vi "Build Wiring Spec.vi"(8 "error in (no error)":errorcluster, 11 "CS++Actor in":refnum<class "CS++Actor.lvclass">) -> (0 "error out":errorcluster, 2 "Wiring Spec":T1, 3 "CS++Actor out":refnum<class "CS++Actor.lvclass">)   [LabVIEW 2016, in "CS++Actor.lvlib" / "CS++Actor.lvclass"]
doc: "Create the Wiring Spec of the original public Vi."
uses:
  CS++Actor.lvclass
  CS++Actor.lvclass/CS++Actor.ctl
  <vilib>/Utility/Data Type/NI_Data Type.lvlib
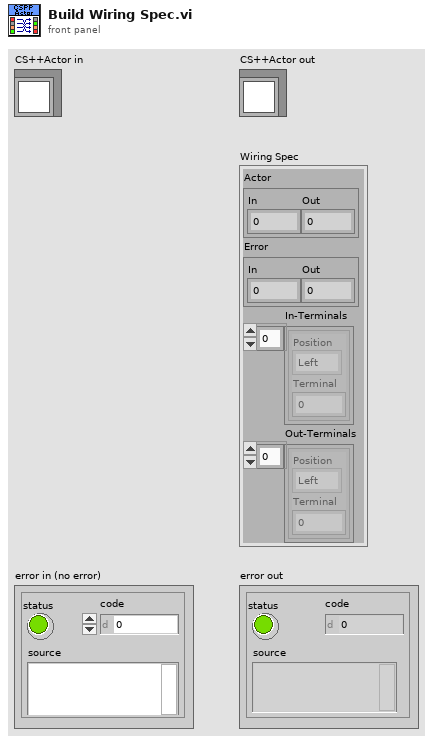
[diagram p1: front panel]
types:
  T1 = cluster{"Actor":cluster{"In":i32, "Out":i32}, "Error":cluster{"In":i32, "Out":i32}, "In-Terminals":cluster{"Position":enum16{"Left", "Top", "Bottom", "Right"}, "Terminal":i32}[], "Out-Terminals":cluster{"Position":enum16{"Left", "Top", "Bottom", "Right"}, "Terminal":i32}[]}
  T2 = cluster{"Actor":cluster{"In":i32, "Out":i32}, "Error":cluster{"In":i32, "Out":i32}, "Left":cluster{"Position":i16, "Terminal":i32}[], "Bottom":cluster{"Position":i16, "Terminal":i32}[], "Right":cluster{"Position":i16, "Terminal":i32}[], "Top":cluster{"Position":i16, "Terminal":i32}[]}
  T3 = enum16{"Invalid Wire Rule", "Required", "Recommended", "Optional", "Dynamic Dispatch"}[]
  T4 = typedef "LVRectTypeDef.ctl" = cluster{"Left":i16, "Top":i16, "Right":i16, "Bottom":i16}
  T5 = cluster{"Position":enum16{"Left", "Top", "Bottom", "Right"}, "Terminal":i32}
  T6 = cluster{"Position":enum16{"Left", "Top", "Bottom", "Right"}, "Terminal":i32}[]
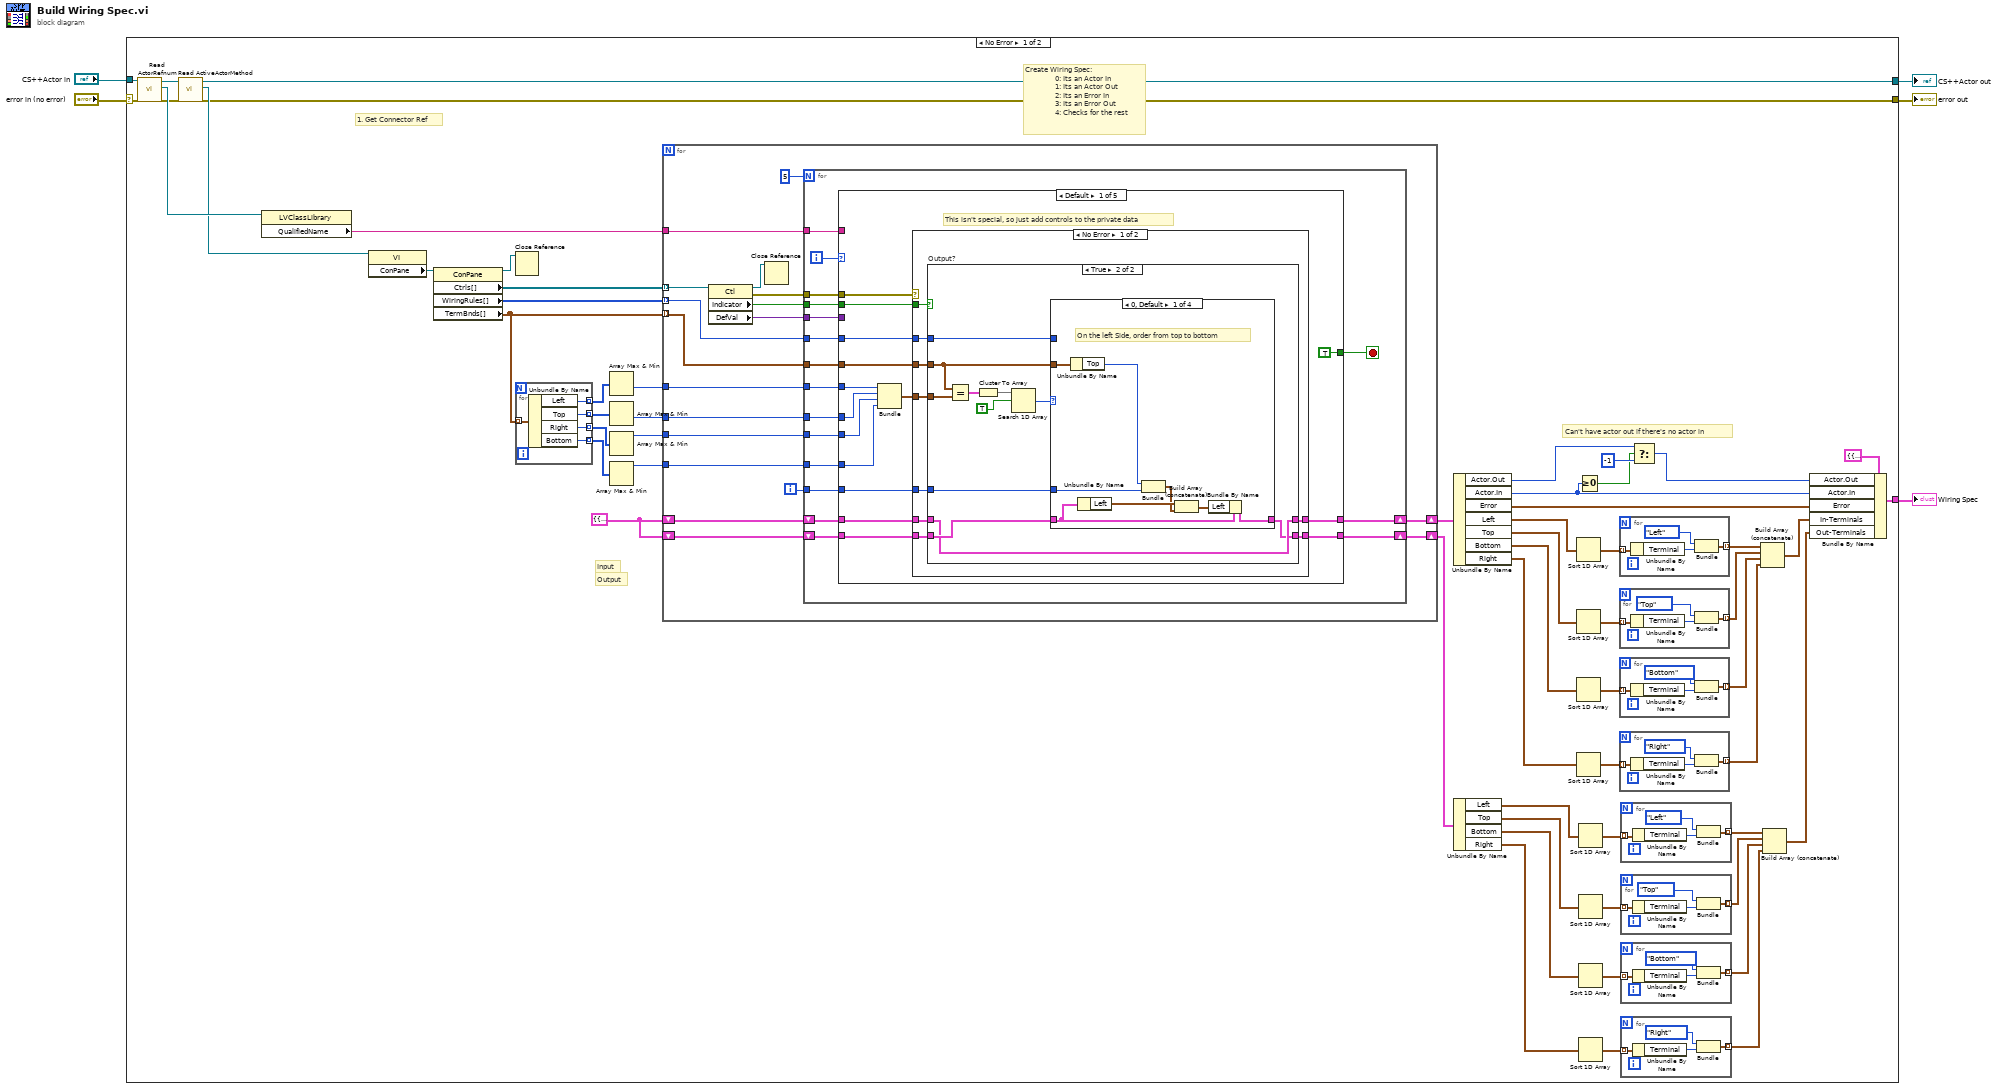
[diagram p0: block diagram]
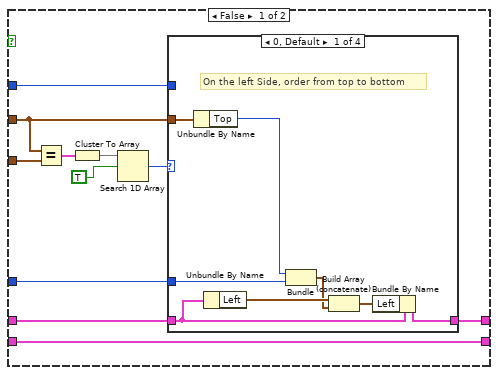
[diagram p2: hidden frame]
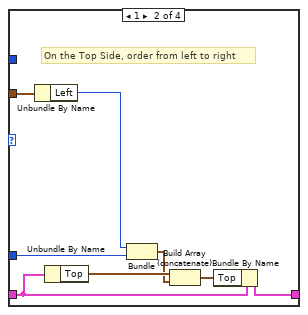
[diagram p3: hidden frame]
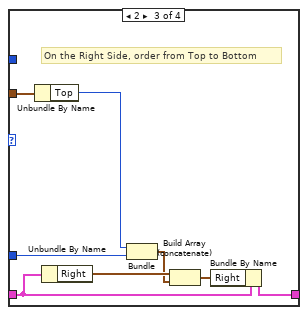
[diagram p4: hidden frame]
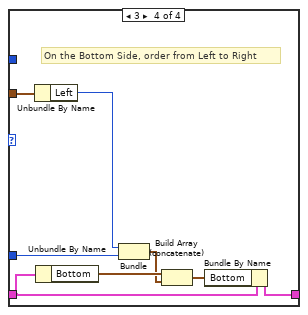
[diagram p5: hidden frame]
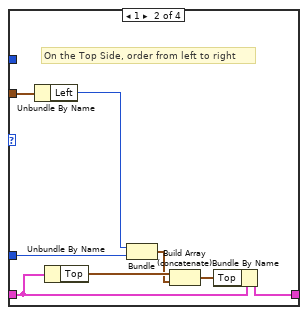
[diagram p6: hidden frame]
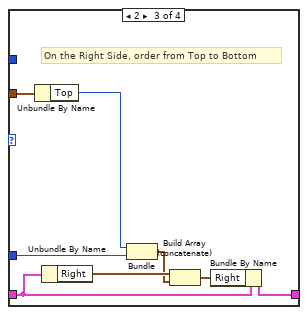
[diagram p7: hidden frame]
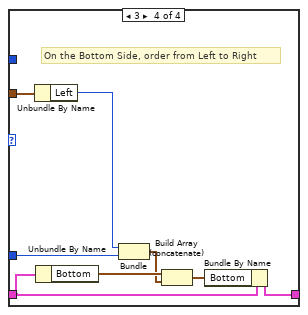
[diagram p8: hidden frame]
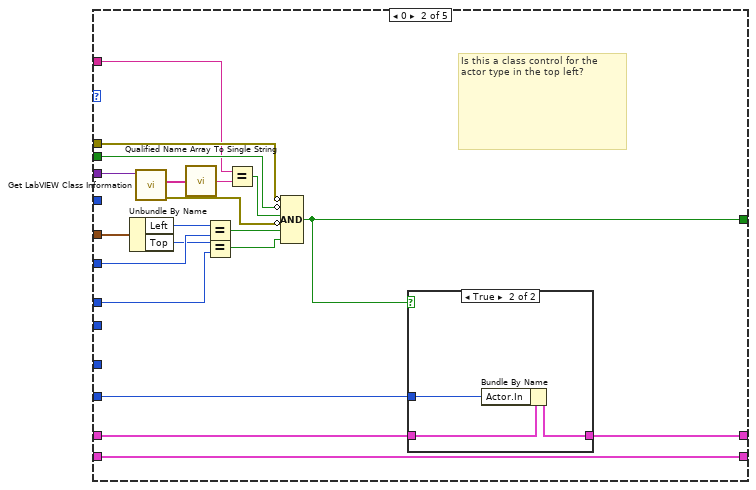
[diagram p10: hidden frame]
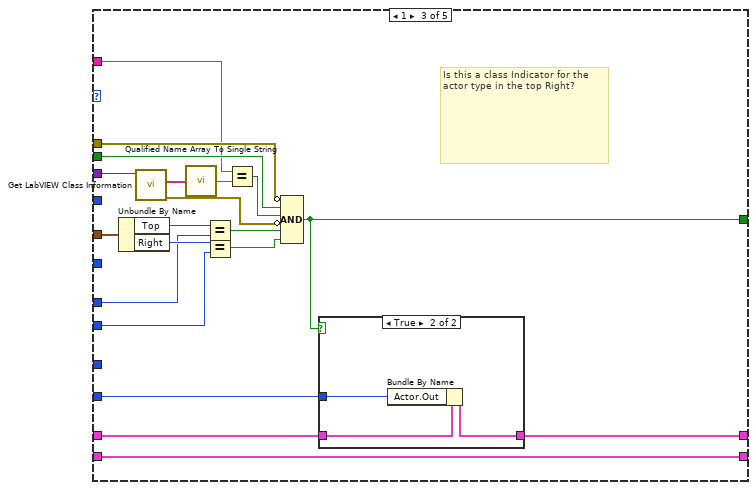
[diagram p12: hidden frame]
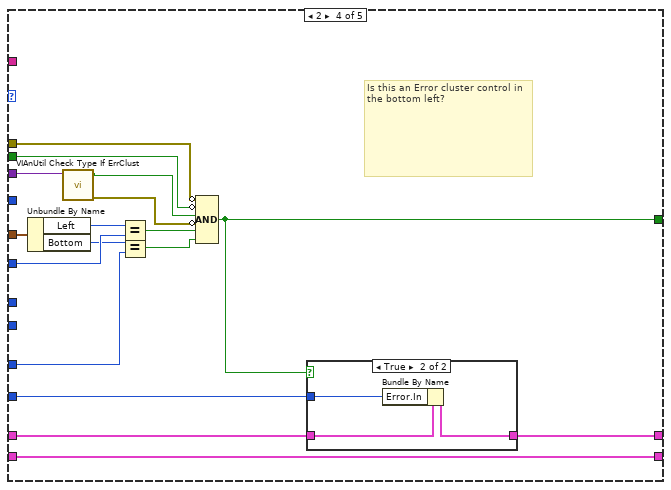
[diagram p14: hidden frame]
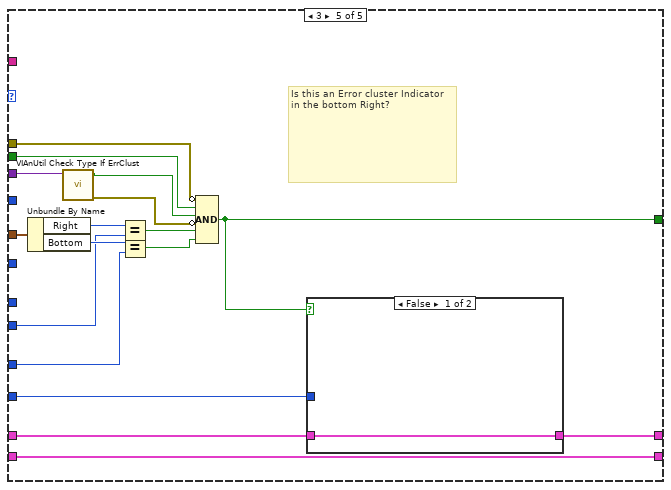
[diagram p16: hidden frame]
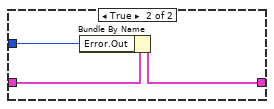
[diagram p17: hidden frame]
diagram:
  n1 = case shown="No Error" "error in (no error)" {
    selector: "error in (no error)" -> [w21 w339]
    tunnel: [w42 _] -> w5
    tunnel: "CS++Actor in" -> [w28 w340]
    tunnel: [w23 w339] -> w3
    tunnel: [w22 w340] -> w2
    frame No Error {
      w20 = T2 {"Actor"={"In"=-1, "Out"=-1}, "Error"={"In"=-1, "Out"=-1}, "Left"=[], "Bottom"=[], "Right"=[], "Top"=[]}
      # "Output"
      # "Input"
      # "Create Wiring Spec:\n               0: Its an Actor In\n               1: Its an Actor Out\n               2: Its an Error In\n               3: Its an Error Out \n               4: Checks for the rest"
      # "1. Get Connector Ref"
      # "Can't have actor out if there's no actor in"
      n2 = call "Read ActorRefnum.vi"("error in (no error)"=w21, "CS++Actor in"=w28) -> ("error out"=w25:errorcluster, "ActorRefnum"=w27:refnum<vi>, "CS++Actor out"=w26:refnum<class "CS++Actor.lvclass">)  [unwired: 7 in]
      n3 = call "Read ActiveActorMethod.vi"("error in (no error)"=w25, "CS++Actor in"=w26) -> ("error out"=w23:errorcluster, "ActiveActorMethod"=w24:refnum<vi>, "CS++Actor out"=w22:refnum<class "CS++Actor.lvclass">)  [unwired: 7 in]
      n4 = property class="LVClassLibrary"(reference=w27) -> ("QualifiedName"=w29:string)  [unwired: 1 in, 2 out]
      n5 = property class="VI"(reference=w24) -> ("ConPane"=w64:refnum<vi>)  [unwired: 1 in, 2 out]
      n6 = property class="ConPane"(reference=w64) -> (reference out=w53:refnum<vi>, "Ctrls[]"=w63:refnum<vi>[], "WiringRules[]"=w41:T3, "TermBnds[]"=w62:T4[])  [unwired: 1 in, 1 out]
      n7 = Close Reference(reference=w53) -> ()  [unwired: 1 in, 1 out]
      n8 = for {
        tunnel: w62 -> [w69] mode=indexing
        tunnel: [w68] -> w61 mode=indexing
        tunnel: [w67] -> w60 mode=indexing
        tunnel: [w66] -> w59 mode=indexing
        tunnel: [w65] -> w58 mode=indexing
        n9 = Unbundle By Name(w69) -> ("Left"=w68:i16, "Top"=w67:i16, "Right"=w66:i16, "Bottom"=w65:i16)
      }
      n10 = Array Max & Min(array=w61) -> (min value=w57:i16)  [unwired: 3 out]
      n11 = Array Max & Min(array=w60) -> (min value=w56:i16)  [unwired: 3 out]
      n12 = Array Max & Min(array=w59) -> (max value=w55:i16)  [unwired: 3 out]
      n13 = Array Max & Min(array=w58) -> (max value=w54:i16)  [unwired: 3 out]
      n14 = for {
        tunnel: w63 -> [w87] mode=indexing
        tunnel: w62 -> [w85] mode=indexing
        tunnel: w57 -> [w84]
        tunnel: w56 -> [w83]
        tunnel: w55 -> [w76]
        tunnel: w54 -> [w77]
        tunnel: w29 -> [w79]
        shift-right: [w73] -> w52
        shift-left: w20 -> [w74]
        tunnel: w41 -> [w72] mode=indexing
        shift-right: [w70] -> w6
        shift-left: w20 -> [w71]
        i -> [w78]
        # "Find Top Left, Bottom left controls AND\nTop Right and bottom right Indicators"
        n15 = property class="Ctl"(reference=w87) -> (reference out=w75:refnum<vi>, error out=w82:errorcluster, "Indicator"=w81:bool, "DefVal"=w80:variant)  [unwired: 1 in]
        n16 = Close Reference(reference=w75) -> ()  [unwired: 1 in, 1 out]
        n17 = for {
          N: 5 -> [_]
          tunnel: w85 -> [w103]
          shift-right: [w94] -> w73
          shift-left: w74 -> [w102]
          tunnel: w84 -> [w101]
          tunnel: w83 -> [w100]
          tunnel: w82 -> [w99]
          tunnel: w81 -> [w98]
          tunnel: w80 -> [w97]
          tunnel: w79 -> [w96]
          tunnel: w78 -> [w95]
          tunnel: w77 -> [w93]
          tunnel: w76 -> [w92]
          tunnel: w72 -> [w90]
          shift-right: [w88] -> w70
          shift-left: w71 -> [w89]
          i -> [w104]
          stop <- w91 stop-if-true
          n18 = case shown="Default" w104 {
            tunnel: w103 -> [w115 w236 w260 w281 w302]
            tunnel: w102 -> [w119 w221 w247 w267 w288]
            tunnel: w101 -> [w114 w234 _ w279 _]
            tunnel: w100 -> [w113 w232 w245 _ _]
            tunnel: w99 -> [w108 w231 w257 w277 w299]
            tunnel: w98 -> [w107 w230 w256 w276 w298]
            tunnel: w97 -> [_ w226 w252 w272 w294]
            tunnel: w96 -> [_ w223 w249 _ _]
            tunnel: w95 -> [w117 w220 w246 w273 w295]
            tunnel: [w118 w218 w242 w266 w287] -> w94
            tunnel: w93 -> [w111 _ _ w269 w291]
            tunnel: w92 -> [w112 _ w244 _ w290]
            tunnel: [TRUE w219 w243 w268 w289] -> w91
            tunnel: w90 -> [w109 _ _ _ _]
            tunnel: w89 -> [w106 w217 w241 w265 w286]
            tunnel: [w105 w217 w241 w265 w286] -> w88
            frame Default {
              # "This isn't special, so just add controls to the private data"
              n19 = Bundle(w114, w113, w112, w111) -> (w110:cluster{i16, i16, i16, i16})  [unwired: 1 in]
              n20 = case shown="No Error" w108 {
                tunnel: w119 -> [w128 w216]
                tunnel: [w127 w216] -> w118
                tunnel: w107 -> [w126 _]
                tunnel: w117 -> [w125 _]
                tunnel: w115 -> [w124 _]
                tunnel: w110 -> [w123 _]
                tunnel: w109 -> [w122 _]
                tunnel: w106 -> [w121 w215]
                tunnel: [w120 w215] -> w105
                frame No Error {
                  n21 = case "Output?" shown="True" w126 {
                    tunnel: w128 -> [w133 w173]
                    tunnel: [w131 w173] -> w127
                    tunnel: w125 -> [w132 w176]
                    tunnel: w124 -> [w134 w177]
                    tunnel: w123 -> [w139 w182]
                    tunnel: w122 -> [w130 w175]
                    tunnel: w121 -> [w129 w174]
                    tunnel: [w129 w172] -> w120
                    frame False {
                      n22 = Equal?(x=w134, y=w139) -> (x = y?=w138:cluster{bool, bool, bool, bool})
                      n23 = Cluster To Array(cluster=w138) -> (array=w137:bool[])
                      n24 = Search 1D Array(1D array=w137, element=TRUE) -> (index of element=w135:i32)  [unwired: 1 in]
                      n25 = case shown="0, Default" w135 {
                        tunnel: w134 -> [w147 w155 w163 w171]
                        tunnel: w133 -> [w144 w152 w160 w168]
                        tunnel: w132 -> [w145 w153 w161 w169]
                        tunnel: [w141 w149 w157 w165] -> w131
                        tunnel: w130 -> [_ _ _ _]
                        frame 0, Default {
                          # "On the left Side, order from top to bottom"
                          n26 = Unbundle By Name(w147) -> ("Top"=w146:i16)
                          n27 = Unbundle By Name(w144) -> ("Left"=w143:cluster{"Position":i16, "Terminal":i32}[])
                          n28 = Bundle("Top"=w146, w145) -> (w142:cluster{"Top":i16, i32})  [unwired: 1 in]
                          n29 = Build Array (concatenate)(w143, w142) -> (w140:cluster{"Top":i16, "Terminal":i32}[])
                          n30 = Bundle By Name(cluster=w144, "Left"=w140) -> (w141:T2)
                        }
                        frame 1 {
                          # "On the Top Side, order from left to right"
                          n31 = Unbundle By Name(w155) -> ("Left"=w154:i16)
                          n32 = Unbundle By Name(w152) -> ("Top"=w151:cluster{"Position":i16, "Terminal":i32}[])
                          n33 = Bundle("Left"=w154, w153) -> (w150:cluster{"Left":i16, i32})  [unwired: 1 in]
                          n34 = Build Array (concatenate)(w151, w150) -> (w148:cluster{"Left":i16, "Terminal":i32}[])
                          n35 = Bundle By Name(cluster=w152, "Top"=w148) -> (w149:T2)
                        }
                        frame 2 {
                          # "On the Right Side, order from Top to Bottom"
                          n36 = Unbundle By Name(w163) -> ("Top"=w162:i16)
                          n37 = Unbundle By Name(w160) -> ("Right"=w159:cluster{"Position":i16, "Terminal":i32}[])
                          n38 = Bundle("Top"=w162, w161) -> (w158:cluster{"Top":i16, i32})  [unwired: 1 in]
                          n39 = Build Array (concatenate)(w159, w158) -> (w156:cluster{"Top":i16, "Terminal":i32}[])
                          n40 = Bundle By Name(cluster=w160, "Right"=w156) -> (w157:T2)
                        }
                        frame 3 {
                          # "On the Bottom Side, order from Left to Right"
                          n41 = Unbundle By Name(w171) -> ("Left"=w170:i16)
                          n42 = Unbundle By Name(w168) -> ("Bottom"=w167:cluster{"Position":i16, "Terminal":i32}[])
                          n43 = Bundle("Left"=w170, w169) -> (w166:cluster{"Left":i16, i32})  [unwired: 1 in]
                          n44 = Build Array (concatenate)(w167, w166) -> (w164:cluster{"Left":i16, "Terminal":i32}[])
                          n45 = Bundle By Name(cluster=w168, "Bottom"=w164) -> (w165:T2)
                        }
                      }
                    }
                    frame True {
                      n46 = Equal?(x=w177, y=w182) -> (x = y?=w181:cluster{bool, bool, bool, bool})
                      n47 = Cluster To Array(cluster=w181) -> (array=w180:bool[])
                      n48 = Search 1D Array(1D array=w180, element=TRUE) -> (index of element=w178:i32)  [unwired: 1 in]
                      n49 = case shown="0, Default" w178 {
                        tunnel: w177 -> [w190 w198 w206 w214]
                        tunnel: w174 -> [w187 w195 w203 w211]
                        tunnel: w176 -> [w188 w196 w204 w212]
                        tunnel: [w184 w192 w200 w208] -> w172
                        tunnel: w175 -> [_ _ _ _]
                        frame 0, Default {
                          # "On the left Side, order from top to bottom"
                          n50 = Unbundle By Name(w190) -> ("Top"=w189:i16)
                          n51 = Unbundle By Name(w187) -> ("Left"=w186:cluster{"Position":i16, "Terminal":i32}[])
                          n52 = Bundle("Top"=w189, w188) -> (w185:cluster{"Top":i16, i32})  [unwired: 1 in]
                          n53 = Build Array (concatenate)(w186, w185) -> (w183:cluster{"Top":i16, "Terminal":i32}[])
                          n54 = Bundle By Name(cluster=w187, "Left"=w183) -> (w184:T2)
                        }
                        frame 1 {
                          # "On the Top Side, order from left to right"
                          n55 = Unbundle By Name(w198) -> ("Left"=w197:i16)
                          n56 = Unbundle By Name(w195) -> ("Top"=w194:cluster{"Position":i16, "Terminal":i32}[])
                          n57 = Bundle("Left"=w197, w196) -> (w193:cluster{"Left":i16, i32})  [unwired: 1 in]
                          n58 = Build Array (concatenate)(w194, w193) -> (w191:cluster{"Left":i16, "Terminal":i32}[])
                          n59 = Bundle By Name(cluster=w195, "Top"=w191) -> (w192:T2)
                        }
                        frame 2 {
                          # "On the Right Side, order from Top to Bottom"
                          n60 = Unbundle By Name(w206) -> ("Top"=w205:i16)
                          n61 = Unbundle By Name(w203) -> ("Right"=w202:cluster{"Position":i16, "Terminal":i32}[])
                          n62 = Bundle("Top"=w205, w204) -> (w201:cluster{"Top":i16, i32})  [unwired: 1 in]
                          n63 = Build Array (concatenate)(w202, w201) -> (w199:cluster{"Top":i16, "Terminal":i32}[])
                          n64 = Bundle By Name(cluster=w203, "Right"=w199) -> (w200:T2)
                        }
                        frame 3 {
                          # "On the Bottom Side, order from Left to Right"
                          n65 = Unbundle By Name(w214) -> ("Left"=w213:i16)
                          n66 = Unbundle By Name(w211) -> ("Bottom"=w210:cluster{"Position":i16, "Terminal":i32}[])
                          n67 = Bundle("Left"=w213, w212) -> (w209:cluster{"Left":i16, i32})  [unwired: 1 in]
                          n68 = Build Array (concatenate)(w210, w209) -> (w207:cluster{"Left":i16, "Terminal":i32}[])
                          n69 = Bundle By Name(cluster=w211, "Bottom"=w207) -> (w208:T2)
                        }
                      }
                    }
                  }
                }
                frame Error {
                }
              }
            }
            frame 0 {
              # "Is this a class control for the actor type in the top left?"
              # "Top Left Actor Class Ctrl?"
              n70 = Unbundle By Name(w236) -> ("Left"=w235:i16, "Top"=w233:i16)
              n71 = call <vilib>:"Get LabVIEW Class Information.vi"("Variant"=w226) -> ("error out"=w225:errorcluster, "Qualified LabVIEW Class Name"=w227:string[])  [unwired: 8 in, 1 out]
              n72 = call <vilib>:"Qualified Name Array To Single String.vi"("Fully Qualified Array"=w227) -> ("Fully Qualified String"=w224:string)
              n73 = Equal?(x=w235, y=w234) -> (x = y?=w229:bool)
              n74 = Equal?(x=w233, y=w232) -> (x = y?=w228:bool)
              n75 = Equal?(x=w223, y=w224) -> (x = y?=w222:bool)
              n76 = Compound Arithmetic op=AND(invert w231, invert w230, w222, invert w225, w229, w228) -> (w219:bool)
              n77 = case shown="True" w219 {
                tunnel: w221 -> [w237 w238]
                tunnel: w220 -> [_ w239]
                tunnel: [w237 w240] -> w218
                frame False {
                }
                frame True {
                  n78 = Bundle By Name(cluster=w238, "Actor.In"=w239) -> (w240:T2)
                }
              }
            }
            frame 1 {
              # "Is this a class Indicator for the actor type in the top Right?"
              # "Top Left Actor Class Ctrl?"
              n79 = Unbundle By Name(w260) -> ("Top"=w259:i16, "Right"=w258:i16)
              n80 = call <vilib>:"Get LabVIEW Class Information.vi"("Variant"=w252) -> ("error out"=w251:errorcluster, "Qualified LabVIEW Class Name"=w253:string[])  [unwired: 8 in, 1 out]
              n81 = call <vilib>:"Qualified Name Array To Single String.vi"("Fully Qualified Array"=w253) -> ("Fully Qualified String"=w250:string)
              n82 = Equal?(x=w259, y=w245) -> (x = y?=w255:bool)
              n83 = Equal?(x=w258, y=w244) -> (x = y?=w254:bool)
              n84 = Equal?(x=w249, y=w250) -> (x = y?=w248:bool)
              n85 = Compound Arithmetic op=AND(invert w257, w256, w248, invert w251, w255, w254) -> (w243:bool)
              n86 = case shown="True" w243 {
                tunnel: w247 -> [w261 w262]
                tunnel: w246 -> [_ w263]
                tunnel: [w261 w264] -> w242
                frame False {
                }
                frame True {
                  n87 = Bundle By Name(cluster=w262, "Actor.Out"=w263) -> (w264:T2)
                }
              }
            }
            frame 2 {
              # "Is this an Error cluster control in the bottom left?"
              # "Top Left Actor Class Ctrl?"
              n88 = Unbundle By Name(w281) -> ("Left"=w280:i16, "Bottom"=w278:i16)
              n89 = call <vilib>:"VIAnUtil Check Type If ErrClust.vi"("Data In"=w272) -> ("error out"=w271:errorcluster, "IsErrClust?"=w270:bool)  [unwired: 9 in]
              n90 = Equal?(x=w280, y=w279) -> (x = y?=w275:bool)
              n91 = Equal?(x=w278, y=w269) -> (x = y?=w274:bool)
              n92 = Compound Arithmetic op=AND(invert w277, invert w276, w270, invert w271, w275, w274) -> (w268:bool)
              n93 = case shown="True" w268 {
                tunnel: w273 -> [_ w284]
                tunnel: [w282 w285] -> w266
                tunnel: w267 -> [w282 w283]
                frame False {
                }
                frame True {
                  n94 = Bundle By Name(cluster=w283, "Error.In"=w284) -> (w285:T2)
                }
              }
            }
            frame 3 {
              # "Is this an Error cluster Indicator in the bottom Right?"
              # "Top Left Actor Class Ctrl?"
              n95 = Unbundle By Name(w302) -> ("Right"=w301:i16, "Bottom"=w300:i16)
              n96 = call <vilib>:"VIAnUtil Check Type If ErrClust.vi"("Data In"=w294) -> ("error out"=w293:errorcluster, "IsErrClust?"=w292:bool)  [unwired: 9 in]
              n97 = Equal?(x=w301, y=w290) -> (x = y?=w297:bool)
              n98 = Equal?(x=w300, y=w291) -> (x = y?=w296:bool)
              n99 = Compound Arithmetic op=AND(invert w299, w298, w292, invert w293, w297, w296) -> (w289:bool)
              n100 = case shown="False" w289 {
                tunnel: w295 -> [_ w305]
                tunnel: [w303 w306] -> w287
                tunnel: w288 -> [w303 w304]
                frame False {
                }
                frame True {
                  n101 = Bundle By Name(cluster=w304, "Error.Out"=w305) -> (w306:T2)
                }
              }
            }
          }
        }
      }
      n102 = Unbundle By Name(w52) -> ("Actor.Out"=w48:i32, "Actor.In"=w45:i32, "Error"=w50:cluster{"In":i32, "Out":i32}, "Left"=w44:cluster{"Position":i16, "Terminal":i32}[], "Top"=w37:cluster{"Position":i16, "Terminal":i32}[], "Bottom"=w36:cluster{"Position":i16, "Terminal":i32}[], "Right"=w35:cluster{"Position":i16, "Terminal":i32}[])
      n103 = Unbundle By Name(w6) -> ("Left"=w10:cluster{"Position":i16, "Terminal":i32}[], "Top"=w9:cluster{"Position":i16, "Terminal":i32}[], "Bottom"=w8:cluster{"Position":i16, "Terminal":i32}[], "Right"=w7:cluster{"Position":i16, "Terminal":i32}[])
      n104 = Sort 1D Array(array=w44) -> (sorted array=w43:cluster{"Position":i16, "Terminal":i32}[])
      n105 = Sort 1D Array(array=w37) -> (sorted array=w40:cluster{"Position":i16, "Terminal":i32}[])
      n106 = Sort 1D Array(array=w36) -> (sorted array=w39:cluster{"Position":i16, "Terminal":i32}[])
      n107 = Sort 1D Array(array=w35) -> (sorted array=w38:cluster{"Position":i16, "Terminal":i32}[])
      n108 = Greater Or Equal To 0?(x=w45) -> (x >= 0?=w46:bool)
      n109 = Sort 1D Array(array=w10) -> (sorted array=w12:cluster{"Position":i16, "Terminal":i32}[])
      n110 = Sort 1D Array(array=w9) -> (sorted array=w13:cluster{"Position":i16, "Terminal":i32}[])
      n111 = Sort 1D Array(array=w8) -> (sorted array=w14:cluster{"Position":i16, "Terminal":i32}[])
      n112 = Sort 1D Array(array=w7) -> (sorted array=w15:cluster{"Position":i16, "Terminal":i32}[])
      n113 = for {
        tunnel: w43 -> [w338] mode=indexing
        tunnel: [w335] -> w34 mode=indexing
        n114 = Unbundle By Name(w338) -> ("Terminal"=w336:i32)
        n115 = Bundle("Position"=enum16{"Left", "Top", "Bottom", "Right"}."Left", "Terminal"=w336) -> (w335:T5)  [unwired: 1 in]
      }
      n116 = for {
        tunnel: w40 -> [w334] mode=indexing
        tunnel: [w331] -> w33 mode=indexing
        n117 = Unbundle By Name(w334) -> ("Terminal"=w332:i32)
        n118 = Bundle("Position"=enum16{"Left", "Top", "Bottom", "Right"}."Top", "Terminal"=w332) -> (w331:T5)  [unwired: 1 in]
      }
      n119 = for {
        tunnel: w39 -> [w330] mode=indexing
        tunnel: [w327] -> w32 mode=indexing
        n120 = Unbundle By Name(w330) -> ("Terminal"=w328:i32)
        n121 = Bundle("Position"=enum16{"Left", "Top", "Bottom", "Right"}."Bottom", "Terminal"=w328) -> (w327:T5)  [unwired: 1 in]
      }
      n122 = for {
        tunnel: w38 -> [w326] mode=indexing
        tunnel: [w323] -> w31 mode=indexing
        n123 = Unbundle By Name(w326) -> ("Terminal"=w324:i32)
        n124 = Bundle("Position"=enum16{"Left", "Top", "Bottom", "Right"}."Right", "Terminal"=w324) -> (w323:T5)  [unwired: 1 in]
      }
      n125 = for {
        tunnel: w12 -> [w322] mode=indexing
        tunnel: [w319] -> w16 mode=indexing
        n126 = Unbundle By Name(w322) -> ("Terminal"=w320:i32)
        n127 = Bundle("Position"=enum16{"Left", "Top", "Bottom", "Right"}."Left", "Terminal"=w320) -> (w319:T5)  [unwired: 1 in]
      }
      n128 = for {
        tunnel: w13 -> [w318] mode=indexing
        tunnel: [w315] -> w17 mode=indexing
        n129 = Unbundle By Name(w318) -> ("Terminal"=w316:i32)
        n130 = Bundle("Position"=enum16{"Left", "Top", "Bottom", "Right"}."Top", "Terminal"=w316) -> (w315:T5)  [unwired: 1 in]
      }
      n131 = for {
        tunnel: w14 -> [w314] mode=indexing
        tunnel: [w311] -> w18 mode=indexing
        n132 = Unbundle By Name(w314) -> ("Terminal"=w312:i32)
        n133 = Bundle("Position"=enum16{"Left", "Top", "Bottom", "Right"}."Bottom", "Terminal"=w312) -> (w311:T5)  [unwired: 1 in]
      }
      n134 = for {
        tunnel: w15 -> [w310] mode=indexing
        tunnel: [w307] -> w19 mode=indexing
        n135 = Unbundle By Name(w310) -> ("Terminal"=w308:i32)
        n136 = Bundle("Position"=enum16{"Left", "Top", "Bottom", "Right"}."Right", "Terminal"=w308) -> (w307:T5)  [unwired: 1 in]
      }
      n137 = Select(t=w48, s=w46, f=-1) -> (s? t:f=w49:i32)
      n138 = Build Array (concatenate)(w34, w33, w32, w31) -> (w30:T6)
      n139 = Build Array (concatenate)(w16, w17, w18, w19) -> (w11:T6)
      n140 = Bundle By Name(cluster=T1 {"Actor"={"In"=0, "Out"=0}, "Error"={"In"=0, "Out"=0}, "In-Terminals"=[], "Out-Terminals"=[]} ("Wiring Spec"), "Actor.Out"=w49, "Actor.In"=w45, "Error"=w50, "In-Terminals"=w30, "Out-Terminals"=w11) -> (w42:T1)
    }
    frame Error {
    }
  }
  "Wiring Spec" <- w5
  "error out" <- w3
  "CS++Actor out" <- w2
